vi "WriteDeviceSettings.vi"(8 "error in (no error)":errorcluster, 10 "Loads":T1[](array[typedef]) {"PowerMax" items=["24 ", "48", "96"]}, 11 "NhRegenGridSim in":refnum<class "NhRegenGridSim.lvclass">) -> (0 "error out":errorcluster, 3 "NhRegenGridSim out":refnum<class "NhRegenGridSim.lvclass">)   [LabVIEW 2018, in "AcPwrPlugins.lvlib" / "NhRegenGridSim.lvclass"]
uses:
  NhRegenGridSim.lvclass
  TypeDefs/DeviceSettings.ctl
  NhRegenGridSim.lvclass/NhRegenGridSim.ctl
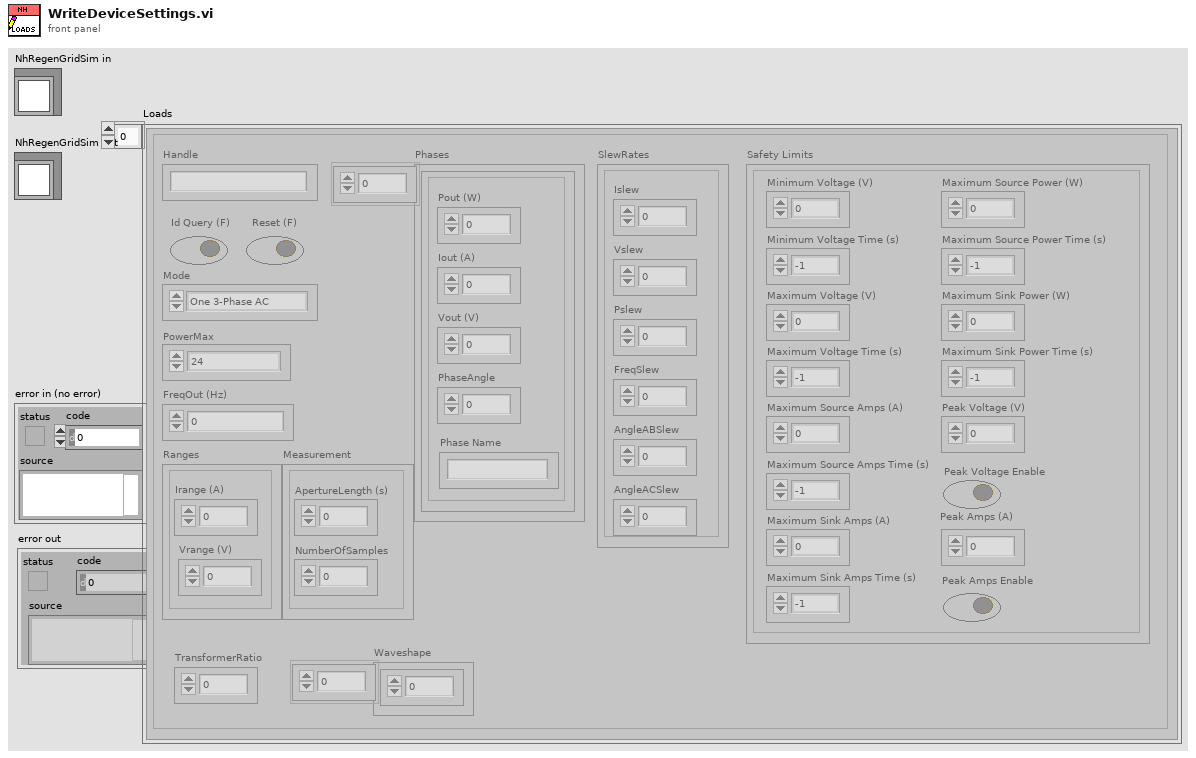
[diagram p1: front panel]
types:
  T1 = typedef "AcPwrPlugins.lvlib/NhRegenGridSim.lvclass/DeviceSettings.ctl" = cluster{"SlewRates":cluster{"Islew":dbl, "Vslew":dbl, "Pslew":dbl, "FreqSlew":dbl, "AngleABSlew":dbl, "AngleACSlew":dbl}, "Phases":cluster{"Pout (W)":dbl, "Iout (A)":dbl, "PhaseAngle":dbl, "Vout (V)":dbl, "Phase Name":string}[], "Measurement":cluster{"ApertureLength (s)":dbl, "NumberOfSamples":u32}, "Ranges":cluster{"Irange (A)":dbl, "Vrange (V)":dbl}, "Mode":enum8{"One 3-Phase AC", "One AC", "One DC", "Three AC", "Three DC", "One 2-Phase AC and One AC", "One 2-Phase AC and One DC", "Two AC", "One AC and One DC", "Two AC and One DC", "One AC and Two DC", "One DC and One AC", "Two DC"}, "PowerMax":u16, "TransformerRatio":dbl, "Waveshape":dbl[], "Handle":string, "FreqOut (Hz)":dbl, "Connected":bool, "Safety Limits":cluster{"Minimum Voltage (V)":dbl, "Minimum Voltage Time (s)":dbl, "Maximum Voltage (V)":dbl, "Maximum Voltage Time (s)":dbl, "Maximum Source Amps (A)":dbl, "Maximum Source Amps Time (s)":dbl, "Maximum Sink Amps (A)":dbl, "Maximum Sink Amps Time (s)":dbl, "Maximum Source Power (W)":dbl, "Maximum Source Power Time (s)":dbl, "Maximum Sink Power (W)":dbl, "Maximum Sink Power Time (s)":dbl, "Peak Voltage (V)":dbl, "Peak Voltage Enable":bool, "Peak Amps (A)":dbl, "Peak Amps Enable":bool}, "btnIdQuery":bool, "btnReset":bool}
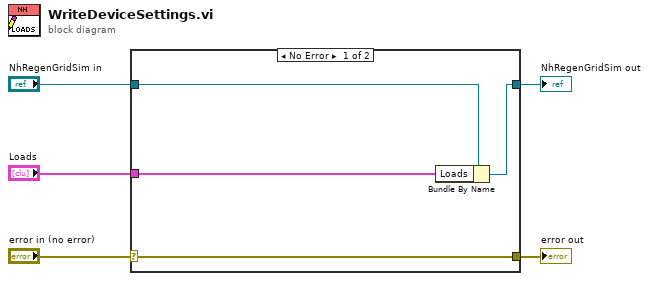
[diagram p0: block diagram]
diagram:
  n1 = case shown="No Error" "error in (no error)" {
    selector: "error in (no error)" -> [w9 w10]
    tunnel: [w9 w10] -> w4
    tunnel: [w7 w11] -> w2
    tunnel: "NhRegenGridSim in" -> [w8 w11]
    tunnel: "Loads" -> [w6 _]
    frame No Error {
      n2 = Bundle By Name(cluster=w8, "Loads"=w6) -> (w7:refnum<class "NhRegenGridSim.lvclass">)
    }
    frame Error {
    }
  }
  "error out" <- w4
  "NhRegenGridSim out" <- w2
